vi "Fill Rect.vi"(8 "error in (no error)":errorcluster, 9 "Colour":u32(colorbox)=16777215, 10 "Rect Pointer":u32 format="%.0x", 11 "Destination Surface Pointer":u32 format="%.0x") -> (0 "error out":errorcluster)   [LabVIEW 2014, in "LibSDL2.lvlib"]
uses:
  LibSDL2.lvlib
  DLL/SDL2.dll
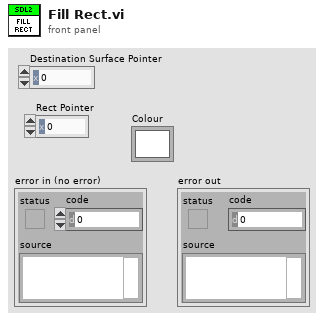
[diagram p1: front panel]
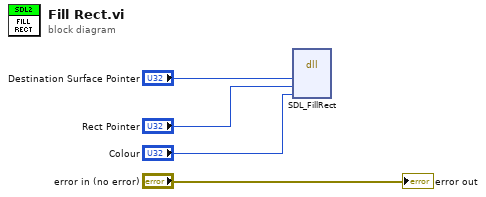
[diagram p0: block diagram]
diagram:
  n1 = dll-call lib="C:/dev/PGS/LabSDL2/Source/LibSDL2 Wrapper/DLL/SDL2.dll" fn="SDL_FillRect"("dst"="Destination Surface Pointer", "rect"="Rect Pointer", "colour"="Colour") -> ()  [unwired: 7 in, 2 out]
  "error out" <- "error in (no error)"
